vi "Get Execution time.vi"(11 "Test Suite Result In":refnum<class "Test Suite Result.lvclass">) -> (3 "Test Suite Result Out":refnum<class "Test Suite Result.lvclass">)   [LabVIEW 2020, in "Test Suite Result.lvclass"]
uses:
  Test Suite Result.lvclass
  Test Suite Result.lvclass/Test Suite Result.ctl
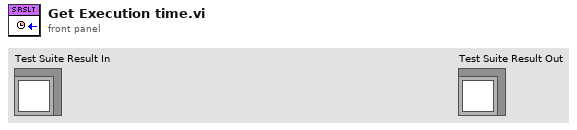
[diagram p1: front panel]
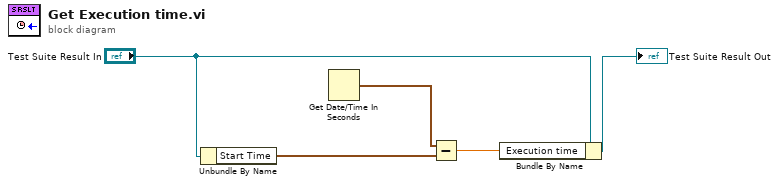
[diagram p0: block diagram]
diagram:
  n1 = Unbundle By Name("Test Suite Result In") -> ("Start Time"=w2:timestamp)
  n2 = Get Date/Time In Seconds() -> (seconds since 1Jan1904=w4:timestamp)
  n3 = Subtract(x=w4, y=w2) -> (x-y=w1:dbl)
  n4 = Bundle By Name(cluster="Test Suite Result In", "Execution time"=w1) -> (→"Test Suite Result Out":refnum<class "Test Suite Result.lvclass">)
